vi "Filter Request.vi"(8 "error in (no error)":errorcluster, 10 "request":refnum<class "request.lvclass">, 11 "Output Actor Hardware in":refnum<class "Output Actor Hardware.lvclass">) -> (0 "error out":errorcluster, 1 "Filtered":bool, 2 "request out":refnum<class "request.lvclass">, 3 "Output Actor Hardware out":refnum<class "Output Actor Hardware.lvclass">)   [LabVIEW 2015, in "Output Actor Hardware.lvclass"]
uses:
  Output Actor Hardware.lvclass
  Request/request.lvclass
  state.ctl
  Output Actor Hardware.lvclass/Output Actor Hardware.ctl
  Output Actor/Output Actor.lvclass
panel:
  in  "state":T1
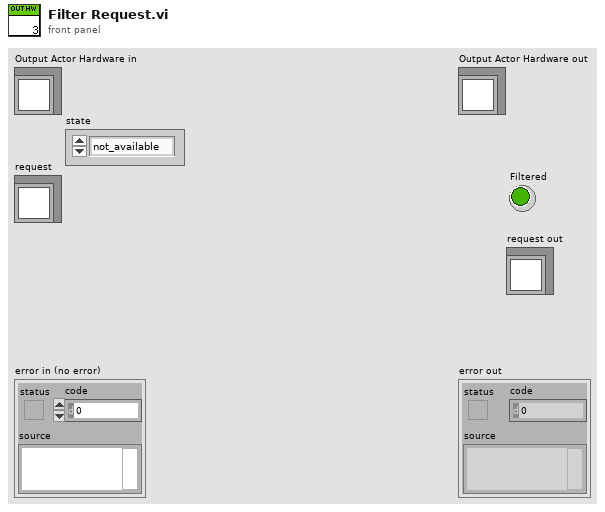
[diagram p1: front panel]
types:
  T1 = typedef "Output Actor Hardware.lvclass/state.ctl" = enum16{"not_available", "not_initialized", "ok"}
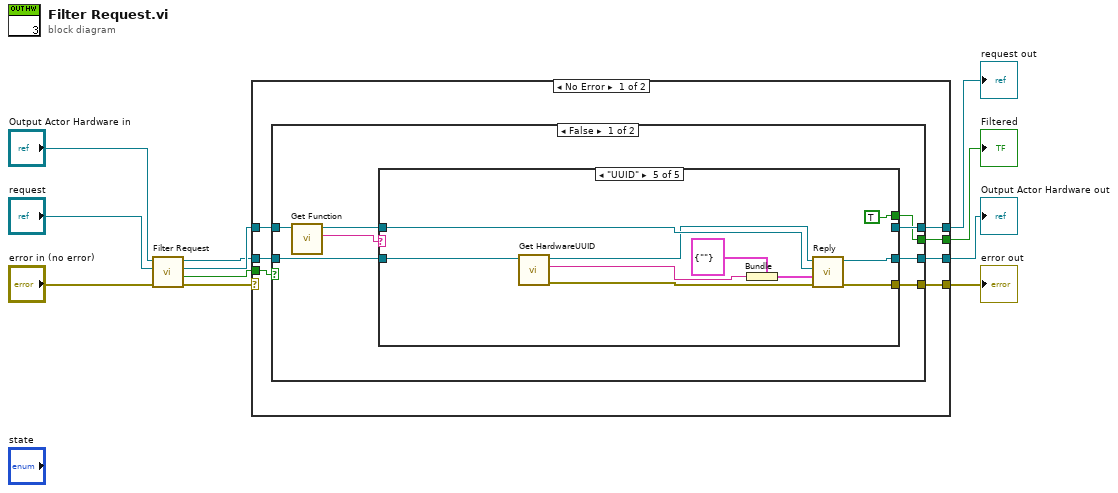
[diagram p0: block diagram]
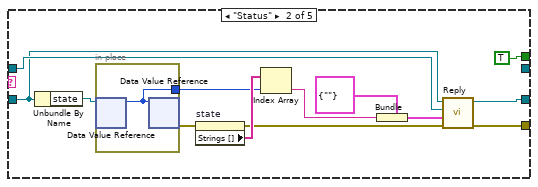
[diagram p3: hidden frame]
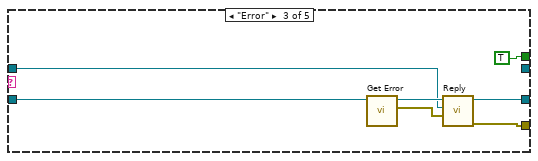
[diagram p4: hidden frame]
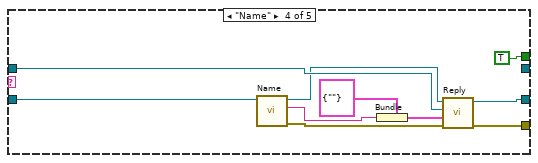
[diagram p5: hidden frame]
diagram:
  n1 = call-parent "Filter Request.vi"("error in (no error)"="error in (no error)", "request"="request", "output_actor in"="Output Actor Hardware in") -> ("error out"=w8:errorcluster, "Filtered"=w7:bool, "request out"=w6:refnum<class "request.lvclass">, "output_actor out"=w3:refnum<class "Output Actor Hardware.lvclass">)  [unwired: 5 in]
  n2 = case shown="No Error" w8 {
    selector: w8 -> [_ w74]
    tunnel: w7 -> [w18 _]
    tunnel: w6 -> [w17 _]
    tunnel: [w12 w74] -> w5
    tunnel: [w16 w73] -> w4
    tunnel: w3 -> [w15 w73]
    tunnel: [w14 _] -> w2
    tunnel: [w13 _] -> w1
    frame No Error {
      n3 = case shown="False" w18 {
        selector: w18 -> [_ w70]
        tunnel: w17 -> [w26 w71]
        tunnel: [w22 w72] -> w16
        tunnel: w15 -> [w21 w72]
        tunnel: [w24 w71] -> w14
        tunnel: [w19 w70] -> w13
        tunnel: [w20 _] -> w12
        frame False {
          n4 = call "Get Function.vi"("request in"=w26) -> ("function"=w25:string, "request out"=w23:refnum<class "request.lvclass">)  [unwired: 8 in, 1 out]
          n5 = case shown="\"UUID\"" w25 {
            tunnel: [w28 _ _ _ _] -> w24
            tunnel: w23 -> [w28 w35 w47 w59 w69]
            tunnel: [w27 w33 w44 w57 w67] -> w22
            tunnel: w21 -> [w27 w34 w49 w53 w63]
            tunnel: [_ w30 w45 w58 w68] -> w20
            tunnel: [_ TRUE TRUE TRUE TRUE] -> w19
            frame "False", Default {
            }
            frame "Status" {
              n6 = Unbundle By Name(w34) -> ("state"=w41:refnum<data-value>)
              n7 = in-place {
                in-place-border: [w42] -> w38
                n8 = in-place-dvr #1(w41) -> (w42:T1)  [unwired: 1 out]
                n9 = in-place-dvr #1(w42) -> (w32:errorcluster)  [unwired: 1 out]
              }
              n10 = property on="state" class="Enum (strict)"(error in=w32) -> (error out=w31:errorcluster, "Strings []"=w39:string[])  [unwired: 1 in, 1 out]
              n11 = Index Array(array=w39, index=w38) -> (element=w37:string)
              n12 = Bundle(cluster=cluster{"Status":string} {"Status"=""}, "Status"=w37) -> (w36:cluster{"Status":string})
              n13 = call "Reply.vi"("error in (no error)"=w31, "Result"=w36, "request"=w35, "output_actor in"=w34) -> ("error out"=w30:errorcluster, "output_actor out"=w33:refnum<class "Output Actor Hardware.lvclass">)  [unwired: 6 in]
            }
            frame "Error" {
              n14 = call "Get Error.vi"("Output Actor Hardware in"=w49) -> ("Error"=w46:errorcluster, "Output Actor Hardware out"=w48:refnum<class "Output Actor Hardware.lvclass">)  [unwired: 8 in, 1 out]
              n15 = call "Reply.vi"("Result"=w46, "request"=w47, "output_actor in"=w48) -> ("error out"=w45:errorcluster, "output_actor out"=w44:refnum<class "Output Actor Hardware.lvclass">)  [unwired: 7 in]
            }
            frame "Name" {
              n16 = call-dynamic "Name.vi"("Output Actor Hardware in"=w53) -> ("error out"=w50:errorcluster, "Name"=w54:string, "Output Actor Hardware out"=w52:refnum<class "Output Actor Hardware.lvclass">)  [unwired: 8 in]
              n17 = Bundle(cluster=cluster{"Name":string} {"Name"=""}, "Name"=w54) -> (w51:cluster{"Name":string})
              n18 = call "Reply.vi"("error in (no error)"=w50, "Result"=w51, "request"=w59, "output_actor in"=w52) -> ("error out"=w58:errorcluster, "output_actor out"=w57:refnum<class "Output Actor Hardware.lvclass">)  [unwired: 6 in]
            }
            frame "UUID" {
              n19 = call "Get HardwareUUID.vi"("Output Actor Hardware in"=w63) -> ("error out"=w60:errorcluster, "UUID"=w61:string, "Output Actor Hardware out"=w62:refnum<class "Output Actor Hardware.lvclass">)  [unwired: 8 in]
              n20 = Bundle(cluster=cluster{"UUID":string} {"UUID"=""}, "UUID"=w61) -> (w64:cluster{"UUID":string})
              n21 = call "Reply.vi"("error in (no error)"=w60, "Result"=w64, "request"=w69, "output_actor in"=w62) -> ("error out"=w68:errorcluster, "output_actor out"=w67:refnum<class "Output Actor Hardware.lvclass">)  [unwired: 6 in]
            }
          }
        }
        frame True {
        }
      }
    }
    frame Error {
    }
  }
  "error out" <- w5
  "Output Actor Hardware out" <- w4
  "request out" <- w2
  "Filtered" <- w1
